vi "Main.vi"() -> ()   [LabVIEW 2018]
uses:
  <vilib>/measure/NI_MABase.lvlib
panel:
  out "Controller Output":dbl
  out "State":dbl
  in  "Schedule":T1(array[cluster])
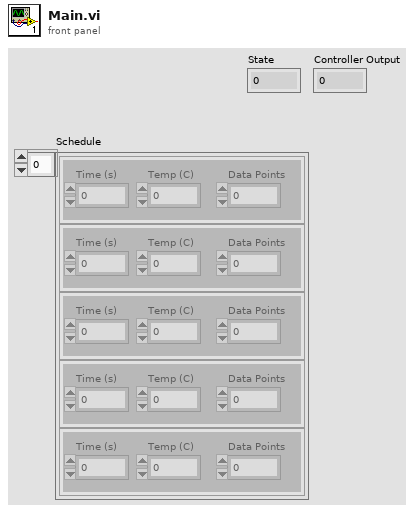
[diagram p1: front panel]
types:
  T1 = cluster{"Time (s)":dbl, "Temp (C)":dbl, "Data Points":dbl}[]
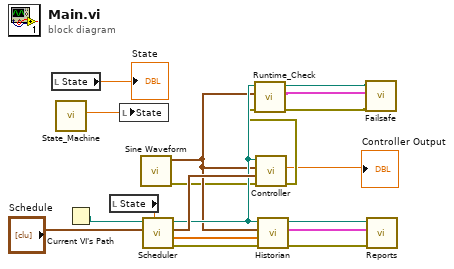
[diagram p0: block diagram]
diagram:
  n1 = local read "State"() -> (→"State":dbl)
  n2 = call "State_Machine.vi"() -> ("State"=w18:dbl)  [unwired: 8 in, 2 out]
  n3 = Current VI's Path() -> (path=w15:path)
  n4 = local read "State"() -> (w16:dbl)
  n5 = local write "State"(w18) -> ()
  n6 = call <vilib>:"Sine Waveform.vi"() -> ("error out"=w3:errorcluster, "signal out"=w7:waveform(dbl))  [unwired: 10 in]
  n7 = call "Scheduler.vi"("Path In"=w15, "Schedule"="Schedule", "Action"=w16) -> ("Path Out"=w8:path, "Mission Stages"=w13:cluster{"Time (s)":dbl, "Temp (C)":dbl}[], "Sampling Rates"=w14:dbl[], "error out"=w12:errorcluster)  [unwired: 4 in]
  n8 = call "Controller.vi"("Path In"=w8, "Signal (Reference)"=w7, "Setpoint Profile"=w13, "error in (no error)"=w3) -> ("Reaction (Output)"=→"Controller Output":dbl, "error out"=w2:errorcluster)  [unwired: 4 in, 1 out]
  n9 = call "Runtime_Check.vi"("error in (no error)"=w2, "Signal"=w7, "Path In"=w8) -> ("error out"=w4:errorcluster, "Outputs"=w5:cluster{"Numeric":dbl, "Boolean":bool}, "Path Out"=w6:path)  [unwired: 5 in, 1 out]
  n10 = call "Historian.vi"("error in (no error)"=w12, "Sampling Rates"=w14, "Sample"=w7, "Path In"=w8) -> ("error out"=w11:errorcluster, "Reports"=w9:cluster{"Numeric":dbl, "Boolean":bool}, "Path Out"=w10:path)  [unwired: 5 in]
  n11 = call "Failsafe.vi"("error in (no error)"=w4, "Inputs"=w5, "Path In"=w6) -> ()  [unwired: 5 in, 4 out]
  n12 = call "Reports.vi"("error in (no error)"=w11, "Inputs"=w9, "Path In"=w10) -> ()  [unwired: 5 in, 4 out]
